vi "Parse Bitfile for EST IP - Multi FPGA.vi"(8 "error in (no error)":errorcluster, 9 "RIO device address":string, 10 "bitfile path":path, 11 "Item Ref in":T1 format="%.0x") -> (0 "error out":errorcluster, 1 "APUs":string[](array[string]), 2 "version":string, 3 "Item Ref out":T1 format="%.0x")   [LabVIEW 2015, in "Engine Simulation Toolkit System Explorer.lvlib"]
uses:
  Engine Simulation Toolkit System Explorer.lvlib
  <vilib>/NI Veristand/Custom Device API/Custom Device Item Ref.ctl
  Shared/Properties.vi
  Shared/Constants and GUIDs.vi
  <vilib>/NI Veristand/Custom Device API/Set Item Property (String).vi
  <vilib>/NI Veristand/Custom Device API/Set Item Property (Boolean).vi
  <vilib>/NI Veristand/Custom Device API/Custom Device API.lvlib
  Shared/Engine Simulation Toolkit Shared.lvlib
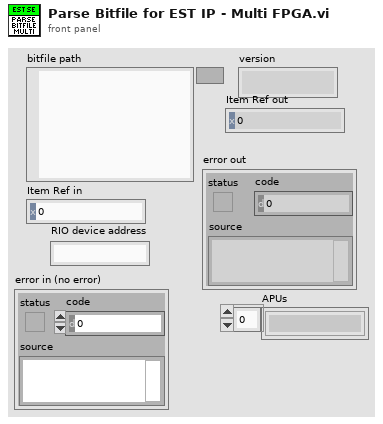
[diagram p1: front panel]
types:
  T1 = typedef "Custom Device API.lvlib/Custom Device Item Ref.ctl" = u64
  T2 = typedef "Engine Simulation Toolkit Shared.lvlib/Bitfile EST Version.ctl" = enum16{"1.0", "1.1", "1.2", "1.3"}
  T3 = typedef "Engine Simulation Toolkit System Explorer.lvlib/String Array Property.ctl" = cluster{"Property Name":string, "Property Value":string[]}
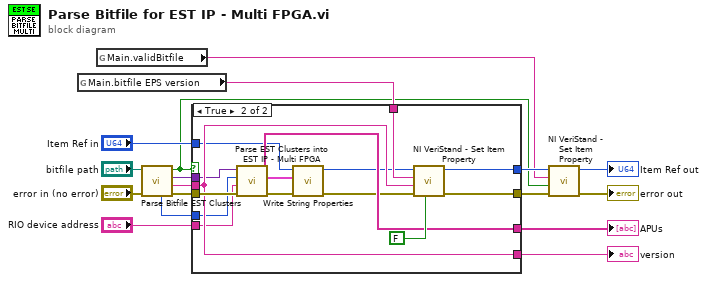
[diagram p0: block diagram]
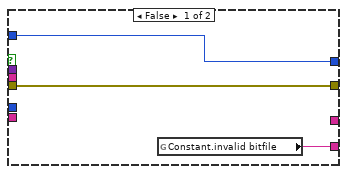
[diagram p2: hidden frame]
diagram:
  n1 = global read "Properties.vi" "Main.bitfile EPS version"() -> (w13:string)
  n2 = global read "Properties.vi" "Main.validBitfile"() -> (w5:string)
  n3 = call "Parse Bitfile EST Clusters.vi"("error in (no error)"="error in (no error)", "bitfile path"="bitfile path") -> ("error out"=w17:errorcluster, "version"=w12:string, "EPS IP LUT"=w15:variant, "valid bitfile"=w4:bool, "EST version enum"=w2:T2)  [unwired: 5 in]
  n4 = case shown="True" w4 {
    tunnel: w17 -> [w20 w35]
    tunnel: w15 -> [_ w28]
    tunnel: "Item Ref in" -> [w19 w23]
    tunnel: w13 -> [_ w34]
    tunnel: w12 -> [_ w31]
    tunnel: [w20 w33] -> w10
    tunnel: [w19 w32] -> w7
    tunnel: [_ w29] -> w9
    tunnel: [w18 w31] -> w3
    tunnel: w2 -> [_ w27]
    tunnel: "RIO device address" -> [_ w21]
    frame False {
      n5 = global read "Constants and GUIDs.vi" "Constant.invalid bitfile"() -> (w18:string)
    }
    frame True {
      n6 = call "Parse EST Clusters into EST IP - Multi FPGA.vi"("error in (no error)"=w35, "RIO device address"=w21, "EST version enum"=w27, "EPS IP LUT"=w28) -> ("error out"=w25:errorcluster, "Properties"=w26:T3[], "APUs"=w29:string[])  [unwired: 5 in]
      n7 = call "Write String Properties.vi"("error in (no error)"=w25, "String Array Properties"=w26, "Item Ref in in"=w23) -> ("error out"=w24:errorcluster, "Item Ref out"=w22:T1)  [unwired: 7 in]
      n8 = call-poly <vilib>:"NI VeriStand - Set Item Property.vi"("Binary String (T)"=FALSE, "error in (no error)"=w24, "Value"=w31, "Property Name"=w34, "Item Ref in"=w22) -> ("error out"=w33:errorcluster, "Item Ref out"=w32:T1)  [unwired: 4 in, 1 out]
    }
  }
  "version" <- w3
  "APUs" <- w9
  n9 = call-poly <vilib>:"NI VeriStand - Set Item Property.vi"("error in (no error)"=w10, "Value"=w4, "Property Name"=w5, "Item Ref in"=w7) -> ("error out"=→"error out":errorcluster, "Item Ref out"=→"Item Ref out":T1)  [unwired: 5 in, 1 out]
